vi "Configure Edge Trigger Source Core.vi"(0 "IVI_Scope in":refnum<class "IVI_Scope.lvclass">, 5 "trigger source (CHANNEL1)":string(combo)="CHANNEL1" caption="trigger source (\"CHANNEL1\")", 7 "trigger slope (Positive)":i32(ring)=1 items=["Positive"=1, "Negative"=0], 9 "trigger level  (0.0 V)":dbl[unit] format="%.3f", 11 "error in (no error)":errorcluster) -> (4 "IVI_Scope out":refnum<class "IVI_Scope.lvclass">, 15 "error out":errorcluster)   [LabVIEW 2016, in "IVI_Scope.lvlib" / "IVI_Scope.lvclass"]
doc: "This VI configures the edge trigger. An edge trigger occurs when the trigger signal passes through the voltage threshold that you specify with the Trigger Level parameter and has the slope that you specify with the Trigger Slope parameter. \n\nNotes:\n (1) This VI affects instrument behavior only if the trigger type is\n IVISCOPE_VAL_EDGE_TRIGGER. Call the IviScope Configure Trigger and\n IviScope Configure Trigger Coupling VIs to set the trigger type and trigger coupling\n before calling this VI.\n (2) If the trigger source is one of the analog input channels, you must configure\n the vertical range, vertical offset, vertical coupling, probe attenuation, and the\n maximum input frequency before calling this VI."
uses:
  IVI_Scope.lvclass
  IVI_Scope.lvclass/IVI_Scope.ctl
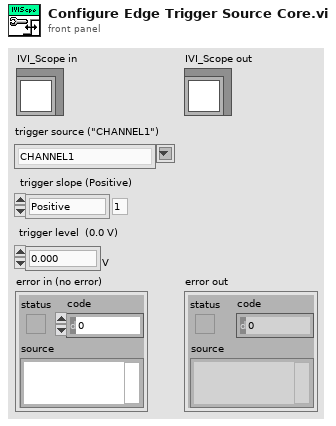
[diagram p1: front panel]
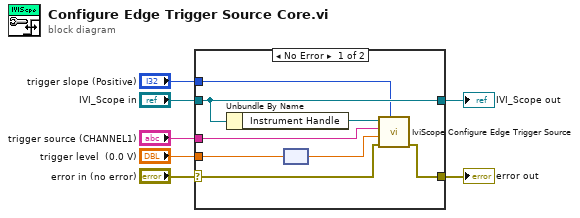
[diagram p0: block diagram]
diagram:
  n1 = case shown="No Error" "error in (no error)" {
    selector: "error in (no error)" -> [w15 w17]
    tunnel: [w14 w17] -> w6
    tunnel: [w13 w16] -> w4
    tunnel: "IVI_Scope in" -> [w13 w16]
    tunnel: "trigger source (CHANNEL1)" -> [w11 _]
    tunnel: "trigger level  (0.0 V)" -> [w10 _]
    tunnel: "trigger slope (Positive)" -> [w9 _]
    frame No Error {
      n2 = Unbundle By Name(w13) -> ("Instrument Handle"=w12:refnum<k15>)
      n3 = node(w10) -> (w8:dbl)
      n4 = call <vilib>:"IviScope Configure Edge Trigger Source.vi"("trigger slope (Positive)"=w9, "error in (no error)"=w15, "trigger level  (0.0 V)"=w8, "trigger source (CHANNEL1)"=w11, "instrument handle"=w12) -> ("error out"=w14:errorcluster)  [unwired: 5 in, 1 out]
    }
    frame Error {
    }
  }
  "error out" <- w6
  "IVI_Scope out" <- w4
